vi "daqmx thermocouples pxi sine test.vi"() -> ()   [LabVIEW 2023]
uses:
  FGen/FGen PXI/FGen PXI Std Waveform CFG/Std Waveform Action Pams.ctl
  Thermometer/Virtual Thermometers/Virt Waveform Reader.lvclass
  Thermometer/Thermometer DAQmx Base CFG/Thermometer DAQmx Base CFG.lvclass
  <vilib>/Waveform/WDTOps.llb/WDT Number of Waveform Samples DBL.vi
  Measure and Stimulus Subsystems/Measure and Stimulus Subsystems.lvclass
  FGen/FGen PXI/FGen PXI Std Waveform CFG.lvlib
panel:
  out "Thermocouple1 Chart":waveform(dbl)(graph)
  in  "Std Waveform Pams":T1={"Frequency"=10.0, "Amplitude"=1.0, "DC Offset"=0.0} {"Frequency" format="%#_g Hz"; "Amplitude" format="%#_g V"; "DC Offset" format="%#_g V"}
  out "total samples fetched":i32
  out "#samples fetched":i32[](array[numeric])
  out "Iteration":i32
  in  "Stop":bool
  out "Error Out":errorcluster
  out "Powersensor Scalar":dbl
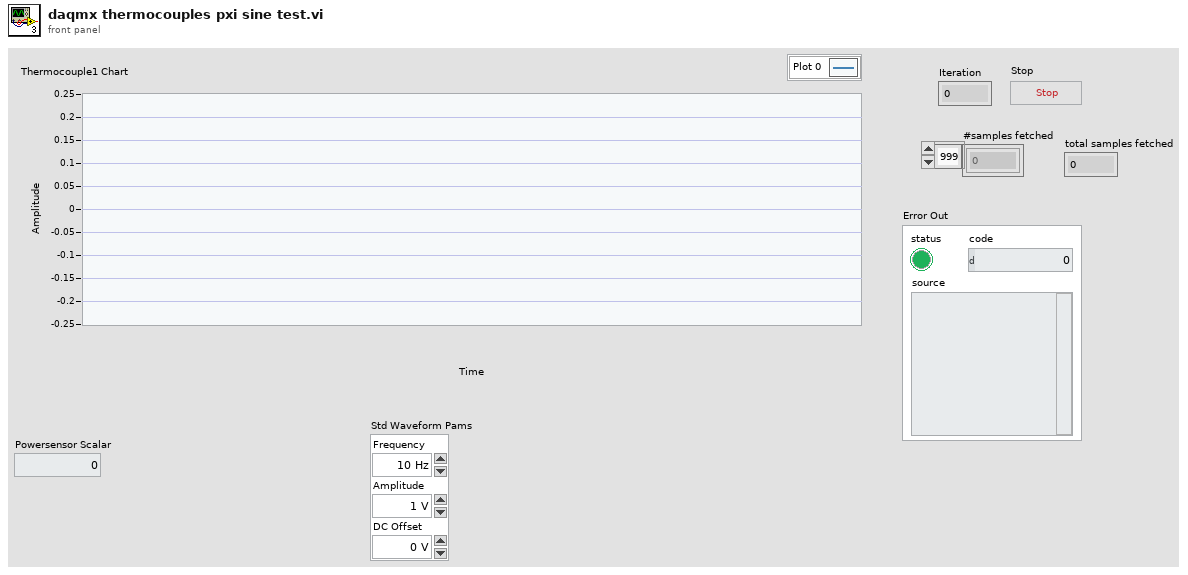
[diagram p1: front panel]
types:
  T1 = typedef "FGen PXI Std Waveform CFG.lvlib/Std Waveform Action Pams.ctl" = cluster{"Frequency":dbl, "Amplitude":dbl, "DC Offset":dbl}
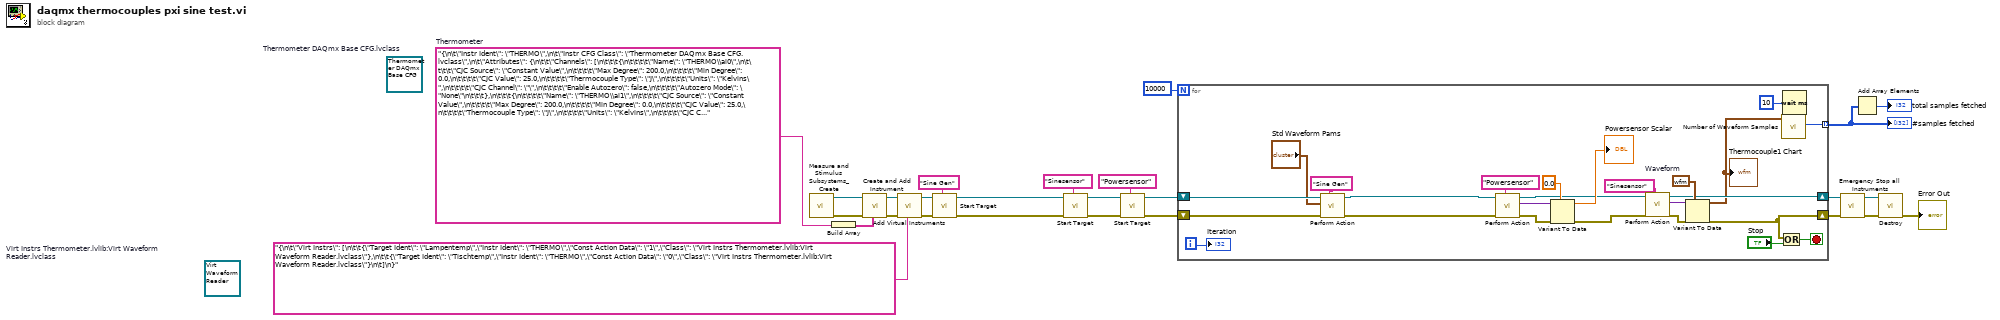
[diagram p0: block diagram]
diagram:
  (unwired) refnum<class "Thermometer DAQmx Base CFG.lvclass"> refnum  # Thermometer DAQmx Base CFG.lvclass
  (unwired) refnum<class "Virt Waveform Reader.lvclass"> refnum  # Virt Instrs Thermometer.lvlib:Virt Waveform Reader.lvclass
  w15 = "{\n\t\"Instr Ident\": \"THERMO\",\n\t\"Instr CFG Class\": \"Thermometer DAQmx Base CFG.lvclass\",\n\t\"Attributes\": {\n\t\t\"Channels\": [\n\t\t\t{\n\t\t\t\t\"Name\": \"THERMO\\ai0\",\n\t\t\t\t\"CJC Source\": \"Constant Value\",\n\t\t\t\t\"Max Degree\": 200.0,\n\t\t\t\t\"Min Degree\": 0.0,\n\t\t\t\t\"CJC Value\": 25.0,\n\t\t\t\t\"Thermocouple Type\": \"J\",\n\t\t\t\t\"Units\": \"Kelvins\",\n\t\t\t\t\"CJC Channel\": \"\",\n\t\t\t\t\"Enable Autozero\": false,\n\t\t\t\t\"Autozero Mode\": \"None\"\n\t\t\t},\n\t\t\t{\n\t\t\t\t\"Name\": \"THERMO\\ai1\",\n\t\t\t\t\"CJC Source\": \"Constant Value\",\n\t\t\t\t\"Max Degree\": 200.0,\n\t\t\t\t\"Min Degree\": 0.0,\n\t\t\t\t\"CJC Value\": 25.0,\n\t\t\t\t\"Thermocouple Type\": \"J\",\n\t\t\t\t\"Units\": \"Kelvins\",\n\t\t\t\t\"CJC Channel\": \"\",\n\t\t\t\t\"Enable Autozero\": false,\n\t\t\t\t\"Autozero Mode\": \"None\"\n\t\t\t},\n\t\t\t{\n\t\t\t\t\"Name\": \"THERMO\\ai2\",\n\t\t\t\t\"CJC Source\": \"Constant Value\",\n\t\t\t\t\"Max Degree\": 200.0,\n\t\t\t\t\"Min Degree\": 0.0,\n\t\t\t\t\"CJC Value\": 25.0,\n\t\t\t\t\"Thermocouple Type\": \"J\",\n\t\t\t\t\"Units\": \"Kelvins\",\n\t\t\t\t\"CJC Channel\": \"\",\n\t\t\t\t\"Enable Autozero\": false,\n\t\t\t\t\"Autozero Mode\": \"None\"\n\t\t\t},\n\t\t\t{\n\t\t\t\t\"Name\": \"THERMO\\ai3\",\n\t\t\t\t\"CJC Source\": \"Constant Value\",\n\t\t\t\t\"Max Degree\": 200.0,\n\t\t\t\t\"Min Degree\": 0.0,\n\t\t\t\t\"CJC Value\": 25.0,\n\t\t\t\t\"Thermocouple Type\": \"J\",\n\t\t\t\t\"Units\": \"Kelvins\",\n\t\t\t\t\"CJC Channel\": \"\",\n\t\t\t\t\"Enable Autozero\": false,\n\t\t\t\t\"Autozero Mode\": \"None\"\n\t\t\t},\n\t\t\t{\n\t\t\t\t\"Name\": \"THERMO\\ai4\",\n\t\t\t\t\"CJC Source\": \"Constant Value\",\n\t\t\t\t\"Max Degree\": 200.0,\n\t\t\t\t\"Min Degree\": 0.0,\n\t\t\t\t\"CJC Value\": 25.0,\n\t\t\t\t\"Thermocouple Type\": \"J\",\n\t\t\t\t\"Units\": \"Kelvins\",\n\t\t\t\t\"CJC Channel\": \"\",\n\t\t\t\t\"Enable Autozero\": false,\n\t\t\t\t\"Autozero Mode\": \"None\"\n\t\t\t},\n\t\t\t{\n\t\t\t\t\"Name\": \"THERMO\\ai5\",\n\t\t\t\t\"CJC Source\": \"Constant Value\",\n\t\t\t\t\"Max Degree\": 200.0,\n\t\t\t\t\"Min Degree\": 0.0,\n\t\t\t\t\"CJC Value\": 25.0,\n\t\t\t\t\"Thermocouple Type\": \"J\",\n\t\t\t\t\"Units\": \"Kelvins\",\n\t\t\t\t\"CJC Channel\": \"\",\n\t\t\t\t\"Enable Autozero\": false,\n\t\t\t\t\"Autozero Mode\": \"None\"\n\t\t\t},\n\t\t\t{\n\t\t\t\t\"Name\": \"THERMO\\ai6\",\n\t\t\t\t\"CJC Source\": \"Constant Value\",\n\t\t\t\t\"Max Degree\": 200.0,\n\t\t\t\t\"Min Degree\": 0.0,\n\t\t\t\t\"CJC Value\": 25.0,\n\t\t\t\t\"Thermocouple Type\": \"J\",\n\t\t\t\t\"Units\": \"Kelvins\",\n\t\t\t\t\"CJC Channel\": \"\",\n\t\t\t\t\"Enable Autozero\": false,\n\t\t\t\t\"Autozero Mode\": \"None\"\n\t\t\t},\n\t\t\t{\n\t\t\t\t\"Name\": \"THERMO\\ai7\",\n\t\t\t\t\"CJC Source\": \"Constant Value\",\n\t\t\t\t\"Max Degree\": 200.0,\n\t\t\t\t\"Min Degree\": 0.0,\n\t\t\t\t\"CJC Value\": 25.0,\n\t\t\t\t\"Thermocouple Type\": \"J\",\n\t\t\t\t\"Units\": \"Kelvins\",\n\t\t\t\t\"CJC Channel\": \"\",\n\t\t\t\t\"Enable Autozero\": false,\n\t\t\t\t\"Autozero Mode\": \"None\"\n\t\t\t}\n\t\t],\n\t\t\"Timing\": {\n\t\t\t\"Samples per Channel\": 1000,\n\t\t\t\"Sample Mode\": \"Continuous Samples\",\n\t\t\t\"Sample Rate\": 10.0,\n\t\t\t\"Sample Clock Source\": \"OnboardClock\",\n\t\t\t\"Active Edge\": \"Rising\",\n\t\t},\n\t\t\"Trigger\": {\n\t\t\t\"Trigger Type\": \"No Trigger\"\n\t\t},\n\t\t\"Acquisition\": {\n\t\t\t\"ReadAllAvailSamp\": True,\n\t\t\t\"Relative To\": \"Current Read Position\",\n\t\t\t\"Overwrite\": \"Do Not Overwrite Unread Samples\",\n\t\t\t\"Samples per Fetch\": 10,\n\t\t\t\"Timeout\": 3.0\n\t\t}\n\t}\n}"  # Thermometer
  n1 = call "Measure and Stimulus Subsystems_Create.vi"() -> ("Error Out"=w25:errorcluster, "reference out"=w26:refnum<class "Measure and Stimulus Subsystems.lvclass">)  [unwired: 10 in]
  n2 = Build Array(w15) -> (w14:string[])
  n3 = call "Create and Add Instrument.vi"("Physical Intr Configs"=w14, "Error In"=w25, "reference in"=w26) -> ("Error Out"=w24:errorcluster, "reference out"=w3:refnum<class "Measure and Stimulus Subsystems.lvclass">)  [unwired: 7 in]
  n4 = call "Add Virtual Instruments.vi"("<JSON CFG>"="{\n\t\"Virt Instrs\": [\n\t\t{\"Target Ident\": \"Lampentemp\",\"Instr Ident\": \"THERMO\",\"Const Action Data\": \"1\",\"Class\": \"Virt Instrs Thermometer.lvlib:Virt Waveform Reader.lvclass\"},\n\t\t{\"Target Ident\": \"Tischtemp\",\"Instr Ident\": \"THERMO\",\"Const Action Data\": \"0\",\"Class\": \"Virt Instrs Thermometer.lvlib:Virt Waveform Reader.lvclass\"}\n\t]\n}", "Error In"=w24, "reference in"=w3) -> ("Error Out"=w4:errorcluster, "reference out"=w2:refnum<class "Measure and Stimulus Subsystems.lvclass">)  [unwired: 7 in]
  n5 = call "Start Target.vi"("Target Ident"="Sine Gen", "Error In"=w4, "reference in"=w2) -> ("Error Out"=w7:errorcluster, "reference out"=w5:refnum<class "Measure and Stimulus Subsystems.lvclass">)  [unwired: 7 in]
  n6 = call "Start Target.vi"("Target Ident"="Sinesensor" ("Target Identifier"), "Error In"=w7, "reference in"=w5) -> ("Error Out"=w17:errorcluster, "reference out"=w10:refnum<class "Measure and Stimulus Subsystems.lvclass">)  [unwired: 7 in]
  n7 = call "Start Target.vi"("Target Ident"="Powersensor", "Error In"=w17, "reference in"=w10) -> ("Error Out"=w11:errorcluster, "reference out"=w9:refnum<class "Measure and Stimulus Subsystems.lvclass">)  [unwired: 7 in]
  n8 = for {
    N: 10000 -> [_]
    shift-right: [w33] -> w19
    shift-left: w11 -> [w49]
    shift-right: [w31] -> w22
    shift-left: w9 -> [w39]
    tunnel: [w40] -> w13 mode=indexing
    i -> [w41]
    stop <- w42 stop-if-true
    w32 = waveform(dbl) {"t0"=timestamp(0 s since 1904-01-01), "dt"=1.0, "Y"=[]}  # Waveform
    n9 = call "Perform Action.vi"("Target Ident"="Sine Gen", "Error In"=w49, "Input"="Std Waveform Pams", "reference in"=w39) -> ("Error Out"=w38:errorcluster, "reference out"=w37:refnum<class "Measure and Stimulus Subsystems.lvclass">)  [unwired: 5 in, 1 out]
    n10 = call "Perform Action.vi"("Target Ident"="Powersensor" ("Target Identifier"), "Error In"=w38, "reference in"=w37) -> ("Error Out"=w50:errorcluster, "Output"=w48:variant, "reference out"=w34:refnum<class "Measure and Stimulus Subsystems.lvclass">)  [unwired: 6 in]
    n11 = Variant To Data(error in=w50, type=0.0, Variant=w48) -> (data=→"Powersensor Scalar":dbl, error out=w43:errorcluster)
    n12 = call "Perform Action.vi"("Target Ident"="Sinesensor", "Error In"=w43, "reference in"=w34) -> ("Error Out"=w29:errorcluster, "Output"=w30:variant, "reference out"=w31:refnum<class "Measure and Stimulus Subsystems.lvclass">)  [unwired: 6 in]
    n13 = Variant To Data(error in=w29, type=w32, Variant=w30) -> (data=w27:waveform(dbl), error out=w33:errorcluster)
    "Thermocouple1 Chart" <- w27
    n14 = Or(x=w33, y="Stop") -> (x .or. y?=w42:bool)
    n15 = call-poly <vilib>:"Number of Waveform Samples.vi"("waveform in"=w27) -> ("number of samples"=w40:i32)  [unwired: 8 in, 2 out]
    n16 = Wait (ms)(milliseconds to wait=u32 10) -> ()  [unwired: 1 out]
    "Iteration" <- w41
  }
  "#samples fetched" <- w13
  n17 = call "Emergency Stop all Instruments.vi"("Error In"=w19, "reference in"=w22) -> ("Error Out"=w23:errorcluster, "reference out"=w21:refnum<class "Measure and Stimulus Subsystems.lvclass">)  [unwired: 8 in]
  n18 = Add Array Elements(numeric array=w13) -> (sum=→"total samples fetched":i32)
  n19 = call "Destroy.vi"("Error In"=w23, "reference in"=w21) -> ("Error Out"=→"Error Out":errorcluster)  [unwired: 8 in, 1 out]
